vi "OE1022_Configure Sensitivity and Filter.vi"(7 "OE1022_Configure Sens and Filter":T1={"Dynamic Reserve"=1, "Sensitivity "=24, "Time Constant "=9, "Low Pass Filter Slope "=1, "Enable Sync Filter "=0} {"Enable Sync Filter" items=["OFF", "ON"]; "Low Pass Filter Slope" items=["6 dB/oct", "12 dB/oct", "18 db/oct", "24 dB/oct"]; "Time Constant" items=["10 us"=1, "30 us"=2, "100 us"=3, "300 us"=4, "1 ms"=5, "3 ms"=6, "10 ms"=7, "30 ms"=8, "100 ms"=9, "300 ms"=10, "1 s"=11, "3 s"=12, "10 s"=13, "30 s"=14, "100 s"=15, "300 s"=16, "1 ks"=17, "3 ks"=18]; "Sensitivity" items=["1 nV/fA"=1, "2 nV/fA"=2, "5 nV/fA"=3, "10 nV/fA"=4, "20 nV/fA"=5, "50 nV/fA"=6, "100 nV/fA"=7, "200 nV/fA"=8, "500 nV/fA"=9, "1 uV/pA"=10, "2 uV/pA"=11, "5 uV/pA"=12, "10 uV/pA"=13, "20 uV/pA"=14, "50 uV/pA"=15, "100 uV/pA"=16, "200 uV/pA"=17, "500 uV/pA"=18, "1 mV/nA"=19, "2 mV/nA"=20, "5 mV/nA"=21, "10 mV/nA"=22, "20 mV/nA"=23, "50 mV/nA"=24, "100 mV/nA"=25, "200 mV/nA"=26, "500 mV/nA"=27, "1 V/uA"=28]; "Dynamic Reserve" items=["Low Noise", "Normal", "High Reserve"]}, 8 "Error in (no error)":errorcluster caption="error out（no error）", 9 "Remote Mode":u16(ring) items=["USB"=0, "GPIB"=2], 11 "VISA resource name":refnum<visa-resource-name>) -> (0 "Error out":errorcluster caption="error out", 1 "Output String":string, 3 "VISA resource  out":refnum<visa-resource-name>)   [LabVIEW 2011]
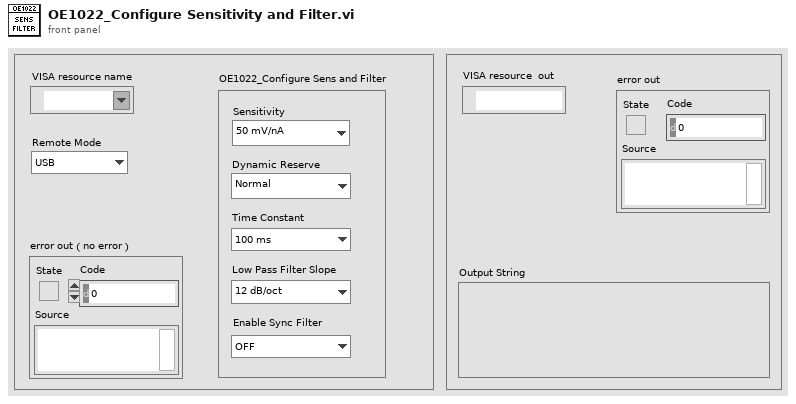
[diagram p1: front panel]
types:
  T1 = cluster{"Dynamic Reserve":u16, "Sensitivity ":u16, "Time Constant ":u8, "Low Pass Filter Slope ":u8, "Enable Sync Filter ":u16}
  T2 = enum16{"ISRC", "IGND", "ICPL", "ILIN", "PHAS", "FMOD", "RSLP", "FREQ", "SWPT", "SLLM", "SULM", "SSLL", "SSLG", "STLM", "SWRM", "IRNG", "SENS", "RMOD", "OFLT", "OFSL", "SYNC", "DMOD", "HARM", "DARB", "SWVT", "SLVL", "SVLL", "SVUL", "SVSL", "SVSG", "SVTM", "SVRM", "RALL", "SNAP", "OUTP", "OAUX", "COUT", "CAUX", "COFP", "CEXP", "FPOP", "OEXP", "*IDN", "*RST", "OVLD", "INOV", "GNOV", "*PLL", "SSET", "RSET", "AGAN", "APHS", "ARSV", "ASCL", "EQCD", "EQCS", "SPED", "SRAT", "SLEN", "SSLE", "STRG", "SPRM", "STRD", "PAUS", "REST", "SPTS", "TRCA", "TEMP", "RSTU", "IHNZ", "DEQU", "SADD", "ARNG", "CSPE", "ISRCD", "IGNDD", "ICPLD", "ILIND", "PHASD", "FMODD", "RSLPD", "FREQD", "SWPTD", "SLLMD", "SULMD", "SSLLD", "SSLGD", "STLMD", "SWRMD", "SENSD", "RMODD", "OFLTD", "OFSLD", "SYNCD", "HARMD", "EQCDD", "EQCSD", "SNAPD", "OUTPD", "SWVTD", "SLVLD", "SVLLD", "SVULD", "SVSLD", "SVSGD", "SVTMD", "SVRMD", "SVDCD", "ARSVD", "AGAND", "APHSD", "ASCLD", "FPOPD", "CAUXD", "OEXPD", "SPEDD", "SRATD", "SLEND", "SSLED", "STRGD", "SPRMD", "STRDD", "PAUSD", "RESTD", "SPTSD", "TRCAD", "*IDND", "*RSTD", "INOVD", "GNOVD", "*PLLD", "SSETD", "RSETD"}
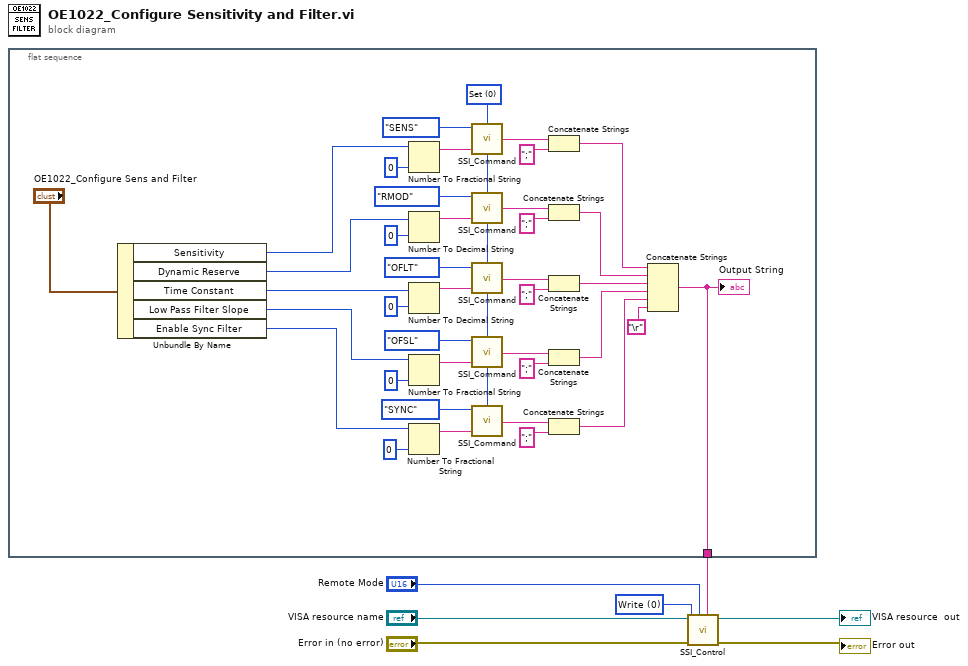
[diagram p0: block diagram]
diagram:
  w6 = u16 0 items=["Write", "Read"] ("Control")
  n1 = flat-sequence {
    tunnel: [w9] -> w1
    frame #0 {
      w17 = u16 0 items=["Set", "Query"] ("Opera")
      n2 = Unbundle By Name("OE1022_Configure Sens and Filter") -> ("Sensitivity"=w27:u16, "Dynamic Reserve"=w26:u16, "Time Constant"=w25:u8, "Low Pass Filter Slope"=w24:u8, "Enable Sync Filter"=w16:u16)
      n3 = Number To Fractional String(number=w27, precision (6)=i16 0 ("精度(6)")) -> (F-format string=w46:string)  [unwired: 2 in]
      n4 = Number To Decimal String(number=w26, width (-)=i16 0 ("宽度(-)")) -> (decimal integer string=w44:string)
      n5 = Number To Decimal String(number=w25, width (-)=i16 0 ("宽度(-)")) -> (decimal integer string=w42:string)
      n6 = Number To Fractional String(number=w24, precision (6)=i16 0 ("精度(6)")) -> (F-format string=w40:string)  [unwired: 2 in]
      n7 = Number To Fractional String(number=w16, precision (6)=i16 0 ("精度(6)")) -> (F-format string=w21:string)  [unwired: 2 in]
      n8 = call "SSI_Command.vi"("Opera"=w17, "Paramter"=w46, "Command Type"=T2."SENS") -> ("Output string"=w33:string)  [unwired: 1 in]
      n9 = call "SSI_Command.vi"("Opera"=w17, "Paramter"=w44, "Command Type"=T2."RMOD") -> ("Output string"=w37:string)  [unwired: 1 in]
      n10 = call "SSI_Command.vi"("Opera"=w17, "Paramter"=w42, "Command Type"=T2."OFLT") -> ("Output string"=w31:string)  [unwired: 1 in]
      n11 = call "SSI_Command.vi"("Opera"=w17, "Paramter"=w40, "Command Type"=T2."OFSL") -> ("Output string"=w35:string)  [unwired: 1 in]
      n12 = call "SSI_Command.vi"("Opera"=w17, "Paramter"=w21, "Command Type"=T2."SYNC") -> ("Output string"=w18:string)  [unwired: 1 in]
      n13 = Concatenate Strings(w33, ";" ("替换字符串(\"\")")) -> (w30:string)
      n14 = Concatenate Strings(w37, ";" ("替换字符串(\"\")")) -> (w29:string)
      n15 = Concatenate Strings(w31, ";" ("替换字符串(\"\")")) -> (w23:string)
      n16 = Concatenate Strings(w35, ";" ("替换字符串(\"\")")) -> (w22:string)
      n17 = Concatenate Strings(w18, ";" ("替换字符串(\"\")")) -> (w10:string)
      n18 = Concatenate Strings(w30, w29, w23, w22, w10, "\r") -> (w9:string)
      "Output String" <- w9
    }
  }
  n19 = call "SSI_Control.vi"("Write Buffer"=w1, "Remote Mode"="Remote Mode", "Error in (no error)"="Error in (no error)", "Control"=w6, "VISA resource name"="VISA resource name") -> ("Error out"=→"Error out":errorcluster, "VISA resource  out"=→"VISA resource  out":refnum<visa-resource-name>)  [unwired: 3 in, 2 out]
